vi "Single Loop Humidity Control.vi"(4 "reinitialize? (F)":bool, 5 "dTmax":dbl=2.0, 6 "dt (s)":dbl=2.0, 7 "PID gains":T1={"proportional gain (Kc)"=2.0, "integral time (Ti, min)"=0.8, "derivative time (Td, min)"=0.0} {"derivative time (Td, min)" format="%.3f"; "integral time (Ti, min)" format="%.3f"; "proportional gain (Kc)" format="%.3f"}, 8 "error in":errorcluster, 9 "TspIn":dbl=2.0, 10 "RHmeas":dbl format="%.2f", 11 "RHsp":dbl format="%.2f") -> (0 "error out":errorcluster, 2 "PID Out":dbl format="%.2f", 3 "TspOut":dbl caption="Td (degC)" format="%.2f")   [LabVIEW 2016]
doc: "This VI updates the temperature setpoint on the UHSAS RH control system using a PID algorithm. For this algortihm:\n* The error, e, is RHsp - RHmeas\n* The output of the control loop is u. This variable is transformed to temperature by associating it with an assumed saturator efficieny. Ideally, the saturator efficiency is 1, but there may be uncertainties that limit this. There fore, the output u, is transformed to an efficiency k by using the following assumptions:\n * when RHmeas < RHsp, k <1\n * when RHmeas > RHsp, k >1\n * when RHmeas = RHsp, k = 1\n To relate temperature to this k, we assume that the k*RHcal= k*esat(Tsp)/esat(Tair)=RHmeas. From this equation, we can calculate the dewpoint of the air exiting the saturator based on the efficiency term k \n* The dewpoint calculated above is the new saturator setpoint."
uses:
  <vilib>/addons/control/pid/pid.llb/PID (DBL).vi
  <vilib>/addons/control/pid/NI_PID_pid.lvlib
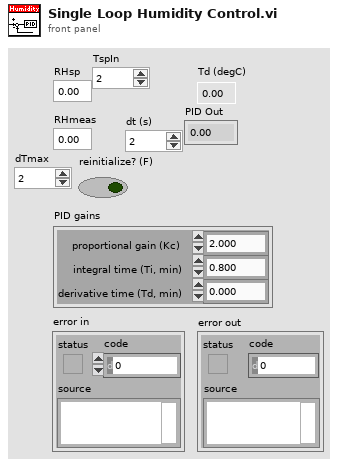
[diagram p1: front panel]
types:
  T1 = cluster{"proportional gain (Kc)":dbl, "integral time (Ti, min)":dbl, "derivative time (Td, min)":dbl}
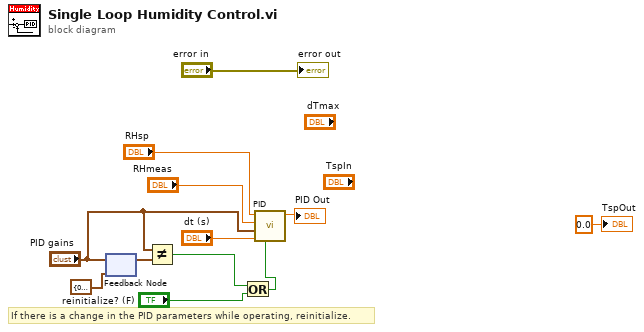
[diagram p0: block diagram]
diagram:
  # "If there is a change in the PID parameters while operating, reinitialize."
  n1 = feedback-in #1("PID gains") -> ()
  n2 = feedback #1(T1 {"proportional gain (Kc)"=0.0, "integral time (Ti, min)"=0.0, "derivative time (Td, min)"=0.0} ("PID gains")) -> (w10:T1)
  n3 = Not Equal?(x="PID gains", y=w10) -> (x != y?=w3:bool)
  n4 = Or(x=w3, y="reinitialize? (F)") -> (x .or. y?=w2:bool)
  n5 = call-poly <vilib>:"PID.vi"("reinitialize? (F)"=w2, "dt (s)"="dt (s)", "PID gains"="PID gains", "process variable"="RHmeas", "setpoint"="RHsp") -> ("output"=→"PID Out":dbl)  [unwired: 5 in, 1 out]
  "error out" <- "error in"
  "TspOut" <- 0.0 ("Tset")
